vi "Motion-Move-X.vi"(4 "X Drive Acc/Speed/Velocity":string="MA1: A 10: V 20: AD 10: D ", 6 "X Coordinates":string="-880000", 8 "error in (no error)":errorcluster, 11 "Motion-ControlAll in":refnum<class "Motion-ControlAll.lvclass">) -> (0 "error out":errorcluster, 3 "Motion-ControlAll out":refnum<class "Motion-ControlAll.lvclass">)   [LabVIEW 2013, in "Motion-ControlAll.lvclass"]
uses:
  Motion-ControlAll.lvclass
  Motion-ControlAll.lvclass/Motion-ControlAll.ctl
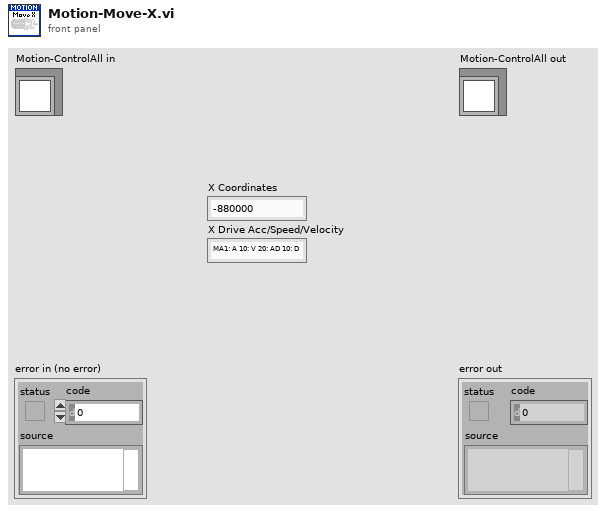
[diagram p1: front panel]
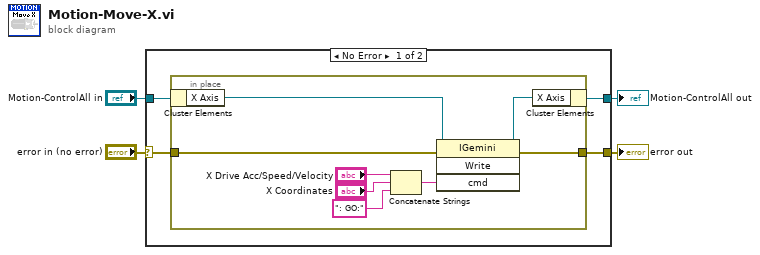
[diagram p0: block diagram]
diagram:
  n1 = case shown="No Error" "error in (no error)" {
    selector: "error in (no error)" -> [w8 w18]
    tunnel: [w7 w18] -> w3
    tunnel: [w6 w17] -> w1
    tunnel: "Motion-ControlAll in" -> [w5 w17]
    frame No Error {
      n2 = in-place {
        in-place-border: w8 -> [w12]
        in-place-border: [w11] -> w7
        n3 = in-place-cluster #1(w5) -> ("X Axis"=w10:refnum<k7>)
        n4 = Concatenate Strings("X Drive Acc/Speed/Velocity", "X Coordinates", ": GO:" ("string")) -> (w13:string)
        n5 = invoke class="IGemini" method="Write"(reference=w10, error in=w12, "cmd"=w13) -> (reference out=w9:refnum<k7>, error out=w11:errorcluster)  [unwired: 1 in, 2 out]
        n6 = in-place-cluster #1("X Axis"=w9) -> (w6:refnum<class "Motion-ControlAll.lvclass">)
      }
    }
    frame Error {
    }
  }
  "error out" <- w3
  "Motion-ControlAll out" <- w1
